vi "rs3 close Sensor.vi"(8 "error in (no error)":errorcluster, 11 "sensor":u64) -> (0 "error out":errorcluster, 2 "device out":u64, 3 "error":u64)   [LabVIEW 2018, in "libRealSense3.lvlib"]
doc: "Close the sensor, after stopping it."
uses:
  libRealSense3.lvlib
  realsense2.dll
panel:
  # "RS3 Close Sensor"
  # "(C) Intel Corp. 2017,  AGJ"
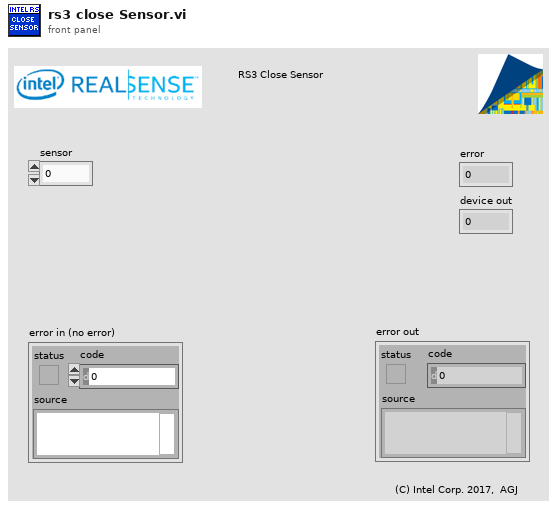
[diagram p1: front panel]
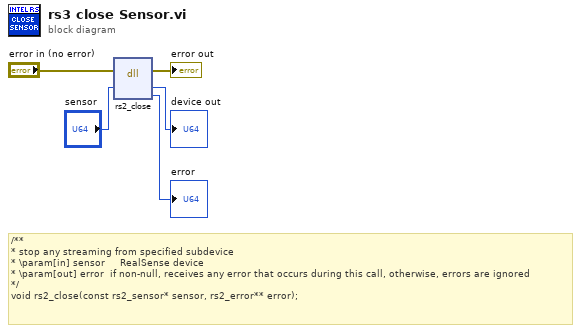
[diagram p0: block diagram]
diagram:
  # "/**\n* stop any streaming from specified subdevice\n* \\param[in] sensor     RealSense device\n* \\param[out] error  if non-null, receives any error that occurs during this call, otherwise, errors are ignored\n*/\nvoid rs2_close(const rs2_sensor* sensor, rs2_error** error);"
  n1 = dll-call lib="C:/Users/aaron.jencks/Documents/Temp/realsense_labview_sdk/RealSense SDK2.11.0 for LabVIEW/realsense2.dll" fn="rs2_close"(error in="error in (no error)", "sensor"="sensor") -> (error out=→"error out":errorcluster, "sensor"=→"device out":u64, "error"=→"error":u64)  [unwired: 4 in, 1 out]
